vi "Foot外观检.vi"() -> ()   [LabVIEW 2022 SP3]
panel:
  out "测试完毕":bool
  out "结果":bool
  in  "Send":bool
  out "error out":errorcluster
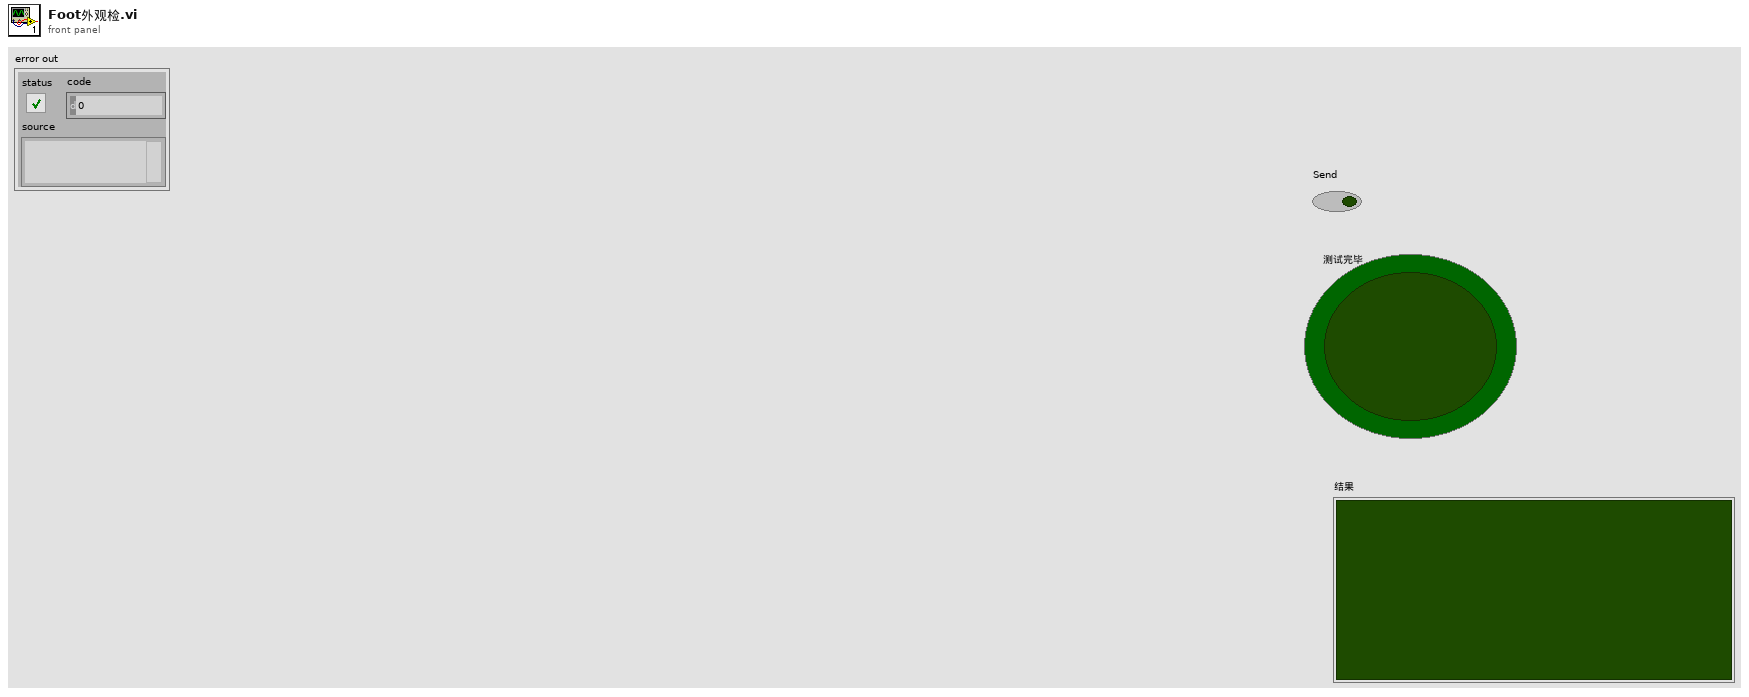
[diagram p1: front panel]
types:
  T1 = typedef "IMAQ Image.ctl" = refnum<image>
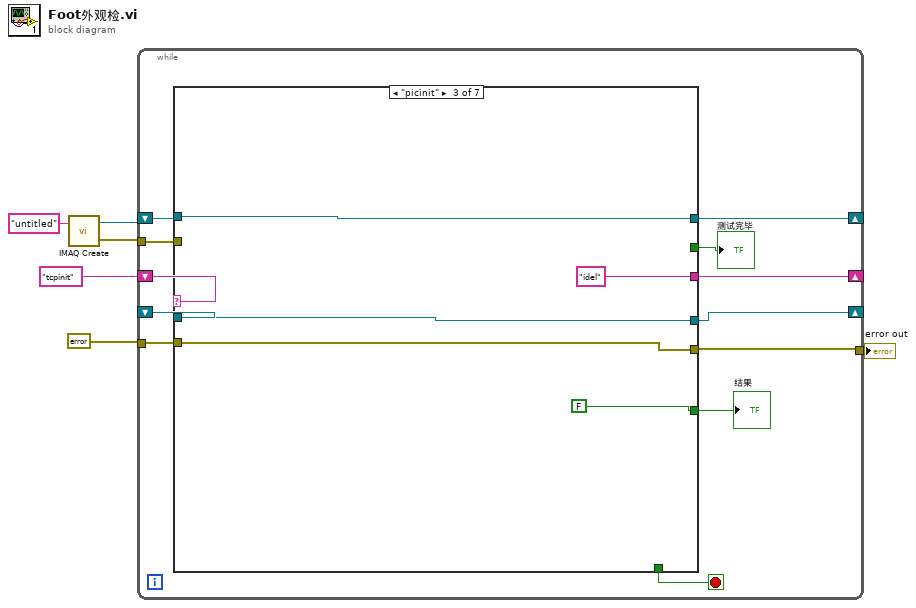
[diagram p0: block diagram]
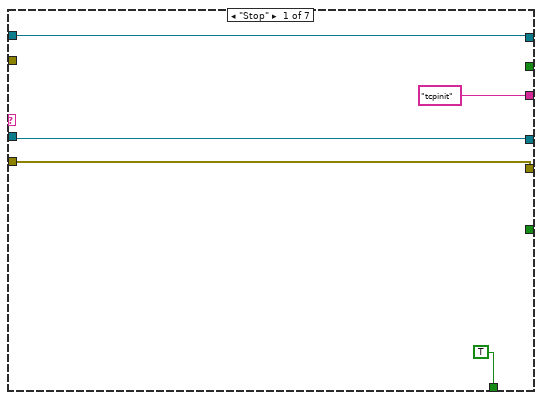
[diagram p2: hidden frame]
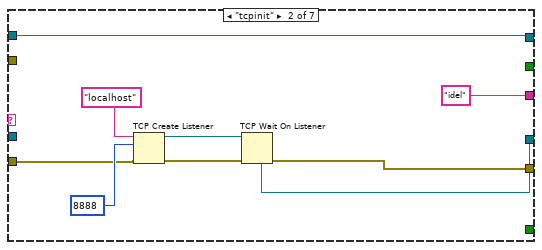
[diagram p3: hidden frame]
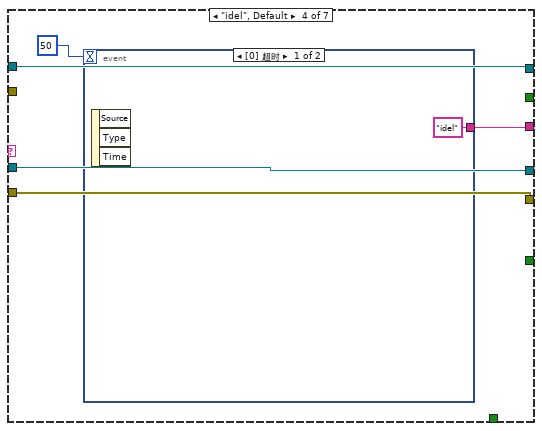
[diagram p4: hidden frame]
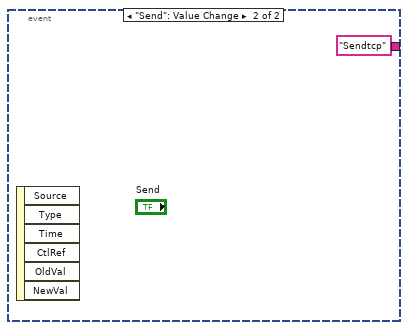
[diagram p5: hidden frame]
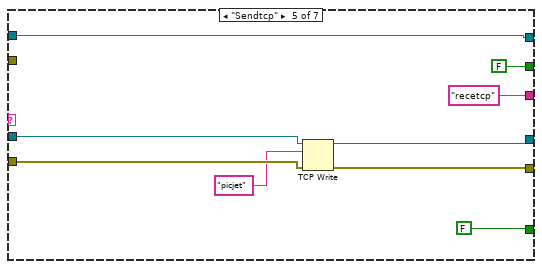
[diagram p6: hidden frame]
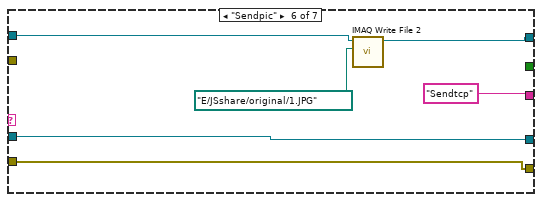
[diagram p7: hidden frame]
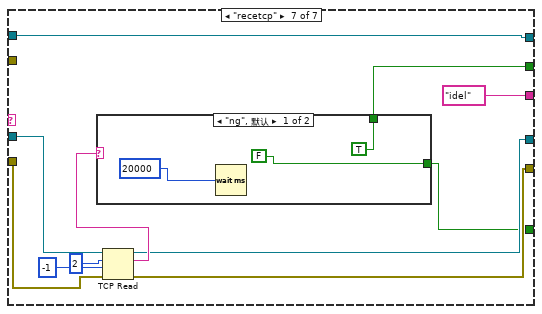
[diagram p8: hidden frame]
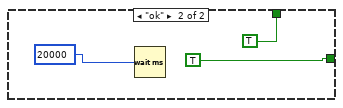
[diagram p9: hidden frame]
diagram:
  n1 = call "IMAQ Create"("Image Name"="untitled") -> ("New Image"=w2:T1, "error out"=w3:errorcluster)  [unwired: 4 in]
  n2 = while {
    shift-right: [w17] -> _
    shift-left: "tcpinit" ("Image Name") -> [w18]
    tunnel: [w16] -> w6
    tunnel: errorcluster {"status"=FALSE, "code"=0, "source"=""} ("error constant") -> [w15]
    shift-right: [w14] -> _
    shift-left: _ -> [w13]
    tunnel: w3 -> [w12]
    shift-right: [w10] -> _
    shift-left: w2 -> [w11]
    stop <- w9 stop-if-true
    n3 = case shown="\"picinit\"" w18 {
      tunnel: ["tcpinit" "idel" "idel" w38 "recetcp" "Sendtcp" "idel"] -> w17
      tunnel: [w20 w30 w37 w40 w51 w55 w63] -> w16
      tunnel: w15 -> [w20 w26 w37 w40 w52 w55 w64]
      tunnel: [w21 w25 w36 w41 w49 w56 w62] -> w14
      tunnel: w13 -> [w21 _ w36 w41 w50 w56 w66]
      tunnel: w11 -> [w22 w24 w34 w42 w53 w59 w70]
      tunnel: w12 -> [_ _ _ _ _ _ _]
      tunnel: [w22 w24 w34 w42 w53 w58 w70] -> w10
      tunnel: [TRUE _ _ _ _ _ _] -> w9
      tunnel: [_ _ _ _ FALSE _ w60] -> w8
      tunnel: [_ _ FALSE _ FALSE _ w61] -> w7
      frame "Stop" {
      }
      frame "tcpinit" {
        n4 = TCP Create Listener(8:w26, 10:u16 8888 ("Port"), 11:"localhost" ("IP Address")) -> (0:w31:errorcluster, 3:w27:refnum<k5>)  [unwired: 2 in, 1 out]
        n5 = TCP Wait On Listener(8:w31, 11:w27) -> (0:w30:errorcluster, 4:w25:refnum<k5>)  [unwired: 2 in, 3 out]
      }
      frame "picinit" {
      }
      frame "idel", Default {
        n6 = event shown="[0] 超时" {
          selector: _ -> [_ _]
          dyn-events: _ -> [_ _]
          timeout: 50 -> [_ _]
          tunnel: ["idel" "Sendtcp"] -> w38
          event Timeout {
            n7 = event-data() -> ()  [unwired: 1 in, 3 out]
          }
          event "Send": Value Change {
            n8 = event-data() -> ()  [unwired: 1 in, 6 out]
          }
        }
      }
      frame "Sendtcp" {
        n9 = TCP Write(connection ID=w50, data in="picjet", error in (no error)=w52) -> (connection ID out=w49:refnum<k5>, error out=w51:errorcluster)  [unwired: 1 in, 1 out]
      }
      frame "Sendpic" {
        n10 = call-poly "IMAQ Write File 2"("File Path"=path "E:/JSshare/original/1.JPG" ("Sent File Path"), "Image"=w59) -> ("Image Out (duplicate)"=w58:T1)  [unwired: 8 in, 1 out]
      }
      frame "recetcp" {
        n11 = TCP Read(connection ID=w66, bytes to read=2, error in (no error)=w64, 9:-1) -> (connection ID out=w62:refnum<k5>, data out=w65:string, error out=w63:errorcluster)  [unwired: 1 out]
        n12 = case shown="\"ng\", 默认" w65 {
          tunnel: [FALSE TRUE] -> w61
          tunnel: [TRUE TRUE] -> w60
          frame "ng", Default {
            n13 = Wait (ms)(milliseconds to wait=20000) -> ()  [unwired: 1 out]
          }
          frame "ok" {
            n14 = Wait (ms)(milliseconds to wait=20000) -> ()  [unwired: 1 out]
          }
        }
      }
    }
    "测试完毕" <- w8
    "结果" <- w7
  }
  "error out" <- w6
